vi "Sonic Straight.vi"   [LabVIEW 2016, in "Test2.lvrbt"]
uses:
  Test2.lvrbt
  <vilib>/NXT/Block Support/NXT_InputPort.ctl
  <vilib>/NXT/Hardware/Plugins/Tetrix DC Motor/TetrixDCMotorAddress.ctl
  <vilib>/NXT/NXTIO Xnodes/NXTIONodeSubVIs/TETRIX IO Move DC Motors.vi
  <vilib>/NXT/Dual Mode Library/Waits/Wait_EV3_Ultrasonic_Centimeter_Closer.vi
  <vilib>/NXT/NXTIO Xnodes/NXTIONodeSubVIs/TETRIX IO Stop DC Motors.vi
  <vilib>/NXT/Dual Mode Library/Waits/Wait_Num.vi
  <vilib>/NXT/Dual Mode Library/Waits/Wait_EV3_Ultrasonic_Centimeters_Further.vi
  <vilib>/NXT/Subs/LVHSConnector.ctl
  <vilib>/NXT/NXTIO Xnodes/AddressXNode/NXTIOAddress.xnode
  <vilib>/NXT/NXTIO Xnodes/NXTIOXNode/NXTIO.xnode
  <vilib>/NXT/LegoClasses/BrickReference/BrickReference.lvclass
types:
  T1 = typedef "NXT_InputPort.ctl" = u32
  T2 = typedef "TetrixDCMotorAddress.ctl" = i32
  T3 = typedef "LVHSConnector.ctl" = refnum<class "BrickReference.lvclass">
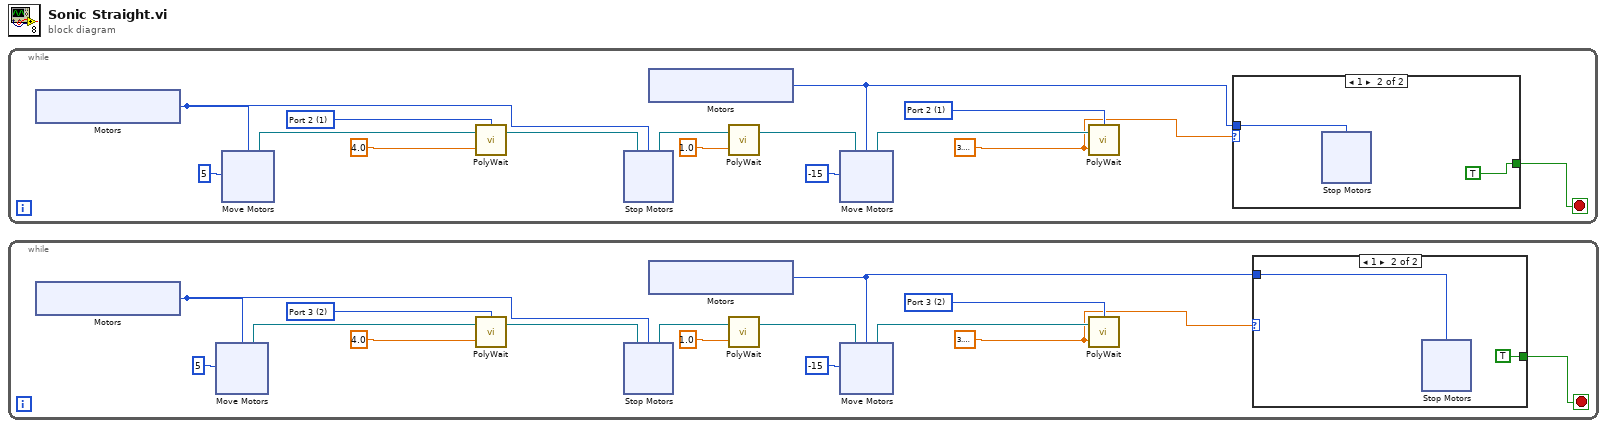
[diagram p0: block diagram]
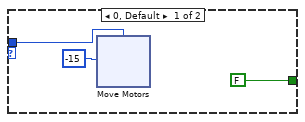
[diagram p2: hidden frame]
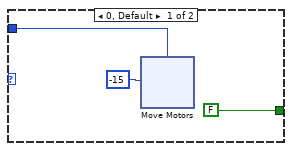
[diagram p3: hidden frame]
diagram:
  n1 = while {
    stop <- w1 stop-if-true
    w4 = T1 1 items=["Port 1", "Port 2", "Port 3", "Port 4"] ("Port (Port 1)")
    w5 = T1 1 items=["Port 1", "Port 2", "Port 3", "Port 4"] ("Port (Port 1)")
    w3 = sgl 3.2 ("Centimeters (50)")
    n2 = xnode "Motors"() -> ("Motor"=w11:T2)
    n3 = xnode "Move Motors"("Power/Speed 1"=i8 5, "Motors"=w11) -> ("NXT/EV3"=w14:T3)  [unwired: 1 in]
    n4 = call-poly <vilib>:"PolyWait.vi"("Centimeters (40)"=sgl 4.0, "NXT/EV3"=w14, "Port (Port 1)"=w5) -> ("NXT/EV3"=w12:T3)  [unwired: 1 in]
    n5 = xnode "Stop Motors"("Motors"=w11, "NXT/EV3"=w12) -> ("NXT/EV3"=w9:T3)
    n6 = xnode "Motors"() -> ("Motor"=w2:T2)
    n7 = call-poly <vilib>:"PolyWait.vi"("Time (1 sec)"=sgl 1.0, "NXT/EV3"=w9) -> ("NXT/EV3"=w8:T3)  [unwired: 2 in]
    n8 = xnode "Move Motors"("Power/Speed 1"=i8 -15, "Motors"=w2, "NXT/EV3"=w8) -> ("NXT/EV3"=w6:T3)
    n9 = call-poly <vilib>:"PolyWait.vi"("Centimeters (50)"=w3, "NXT/EV3"=w6, "Port (Port 1)"=w4) -> ()  [unwired: 1 in, 1 out]
    n10 = case shown="1" w3 {
      tunnel: w2 -> [w16 w27]
      tunnel: [FALSE TRUE] -> w1
      frame 0, Default {
        n11 = xnode "Move Motors"("Power/Speed 1"=i8 -15, "Motors"=w16) -> ()  [unwired: 1 in, 1 out]
      }
      frame 1 {
        n12 = xnode "Stop Motors"("Motors"=w27) -> ()  [unwired: 1 in, 1 out]
      }
    }
  }
  n13 = while {
    stop <- w55 stop-if-true
    w57 = T1 2 items=["Port 1", "Port 2", "Port 3", "Port 4"] ("Port (Port 1)")
    w58 = T1 2 items=["Port 1", "Port 2", "Port 3", "Port 4"] ("Port (Port 1)")
    w54 = sgl 3.2 ("Centimeters (50)")
    n14 = xnode "Motors"() -> ("Motor"=w56:T2)
    n15 = xnode "Move Motors"("Power/Speed 1"=i8 5, "Motors"=w56) -> ("NXT/EV3"=w67:T3)  [unwired: 1 in]
    n16 = call-poly <vilib>:"PolyWait.vi"("Centimeters (40)"=sgl 4.0, "NXT/EV3"=w67, "Port (Port 1)"=w58) -> ("NXT/EV3"=w65:T3)  [unwired: 1 in]
    n17 = xnode "Stop Motors"("Motors"=w56, "NXT/EV3"=w65) -> ("NXT/EV3"=w63:T3)
    n18 = xnode "Motors"() -> ("Motor"=w59:T2)
    n19 = call-poly <vilib>:"PolyWait.vi"("Time (1 sec)"=sgl 1.0, "NXT/EV3"=w63) -> ("NXT/EV3"=w62:T3)  [unwired: 2 in]
    n20 = xnode "Move Motors"("Power/Speed 1"=i8 -15, "Motors"=w59, "NXT/EV3"=w62) -> ("NXT/EV3"=w60:T3)
    n21 = call-poly <vilib>:"PolyWait.vi"("Centimeters (50)"=w54, "NXT/EV3"=w60, "Port (Port 1)"=w57) -> ()  [unwired: 1 in, 1 out]
    n22 = case shown="1" w54 {
      tunnel: w59 -> [w69 w80]
      tunnel: [FALSE TRUE] -> w55
      frame 0, Default {
        n23 = xnode "Move Motors"("Power/Speed 1"=i8 -15, "Motors"=w69) -> ()  [unwired: 1 in, 1 out]
      }
      frame 1 {
        n24 = xnode "Stop Motors"("Motors"=w80) -> ()  [unwired: 1 in, 1 out]
      }
    }
  }
